vi "VI Tree.vi"   [LabVIEW 2013, in "Counter.lvlib" / "PICOTEST U62XXA series.lvlib"]
doc: "This is the instrument driver for the PICOTEST U62XXA series. The VI Tree displays all the user-callable VIs of the instrument driver in an organized table."
uses:
  PICOTEST U62XXA series.lvlib
  Configure/Configure Arming (Auto).vi
  Data/Read (Measurement).vi
  Data/Low level Data/Fetch (Measurement).vi
panel:
  # "(c) 2009 PICOTEST CORP  ALL RIGHTS RESERVED."
  # "SEE DIAGRAM\nFOR VI TREE."
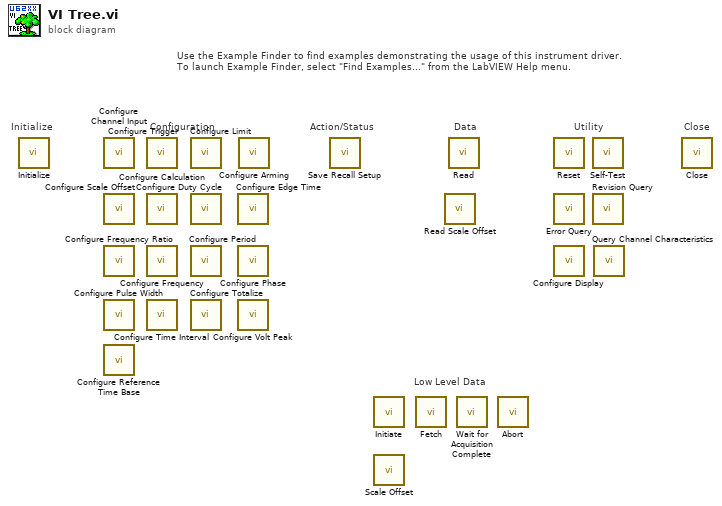
[diagram p0: block diagram]
diagram:
  # "Low Level Data"
  # "Use the Example Finder to find examples demonstrating the usage of this instrument driver.\nTo launch Example Finder, select \"Find Examples...\" from the LabVIEW Help menu."
  # "Configuration"
  # "Utility"
  # "Data"
  # "Action/Status"
  # "Close"
  # "Initialize"
  n1 = call "Initialize.vi"() -> ()  [unwired: 9 in, 3 out]
  n2 = call "Configure Channel Input.vi"() -> ()  [unwired: 10 in, 2 out]
  n3 = call "Configure Scale Offset.vi"() -> ()  [unwired: 10 in, 2 out]
  n4 = call "Configure Frequency Ratio.vi"() -> ()  [unwired: 10 in, 2 out]
  n5 = call "Configure Pulse Width.vi"() -> ()  [unwired: 10 in, 2 out]
  n6 = call "Configure Reference Time Base.vi"() -> ()  [unwired: 10 in, 2 out]
  n7 = call "Configure Trigger.vi"() -> ()  [unwired: 10 in, 2 out]
  n8 = call "Configure Calculation.vi"() -> ()  [unwired: 10 in, 2 out]
  n9 = call "Configure Frequency.vi"() -> ()  [unwired: 10 in, 2 out]
  n10 = call "Configure Time Interval.vi"() -> ()  [unwired: 10 in, 2 out]
  n11 = call "Configure Limit.vi"() -> ()  [unwired: 10 in, 2 out]
  n12 = call "Configure Duty Cycle.vi"() -> ()  [unwired: 10 in, 2 out]
  n13 = call "Configure Period.vi"() -> ()  [unwired: 10 in, 2 out]
  n14 = call "Configure Totalize.vi"() -> ()  [unwired: 10 in, 2 out]
  n15 = call "Configure Edge Time.vi"() -> ()  [unwired: 10 in, 2 out]
  n16 = call "Configure Phase.vi"() -> ()  [unwired: 10 in, 2 out]
  n17 = call "Configure Volt Peak.vi"() -> ()  [unwired: 10 in, 2 out]
  n18 = call-poly "Configure Arming.vi"() -> ()  [unwired: 14 in, 2 out]
  n19 = call "Save Recall Setup.vi"() -> ()  [unwired: 10 in, 2 out]
  n20 = call "Initiate.vi"() -> ()  [unwired: 10 in, 2 out]
  n21 = call "Scale Offset.vi"() -> ()  [unwired: 9 in, 3 out]
  n22 = call-poly "Fetch.vi"() -> ()  [unwired: 9 in, 3 out]
  n23 = call "Read Scale Offset.vi"() -> ()  [unwired: 9 in, 3 out]
  n24 = call-poly "Read.vi"() -> ()  [unwired: 9 in, 3 out]
  n25 = call "Wait for Acquisition Complete.vi"() -> ()  [unwired: 10 in, 2 out]
  n26 = call "Abort.vi"() -> ()  [unwired: 10 in, 2 out]
  n27 = call "Reset.vi"() -> ()  [unwired: 10 in, 2 out]
  n28 = call "Error Query.vi"() -> ()  [unwired: 8 in, 4 out]
  n29 = call "Configure Display.vi"() -> ()  [unwired: 10 in, 2 out]
  n30 = call "Self-Test.vi"() -> ()  [unwired: 8 in, 4 out]
  n31 = call "Revision Query.vi"() -> ()  [unwired: 8 in, 4 out]
  n32 = call "Query Channel Characteristics.vi"() -> ()  [unwired: 5 in, 7 out]
  n33 = call "Close.vi"() -> ()  [unwired: 11 in, 1 out]
